vi "lantronix_discovery.vi"(8 "error in (no error)":errorcluster, 10 "timeout [ms] (1000)":dbl=1.0 caption="timeout [ms]", 11 "Local IP (optional)":string) -> (0 "error out":errorcluster, 3 "DEVICES":T1(array[cluster]))   [LabVIEW 2016]
doc: "This VI scans network and tries to find all connected Lantronix X-Port devices.\nThe result is array of clusters of 4 elements (IP, MAC, ID, version).\nUser can enter valid Local IP Address or this vi tries to get local IP from system.\n\nJakub Parez ATEsystem s.r.o. 2017"
uses:
  <vilib>/Utility/error.llb/Error Cluster From Error Code.vi
  <vilib>/regexp/Match Regular Expression.xnode
  <vilib>/ErrorRing/Error Ring.xnode
panel:
  # "IP"
  # "MAC"
  # "ID"
  # "version"
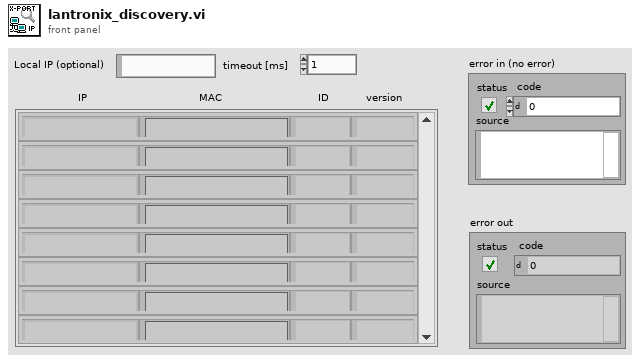
[diagram p1: front panel]
types:
  T1 = cluster{"IP":string, "MAC":string, "ID":string, "version":string}[]
  T2 = cluster{"IP":string, "MAC":string, "ID":string, "version":string}
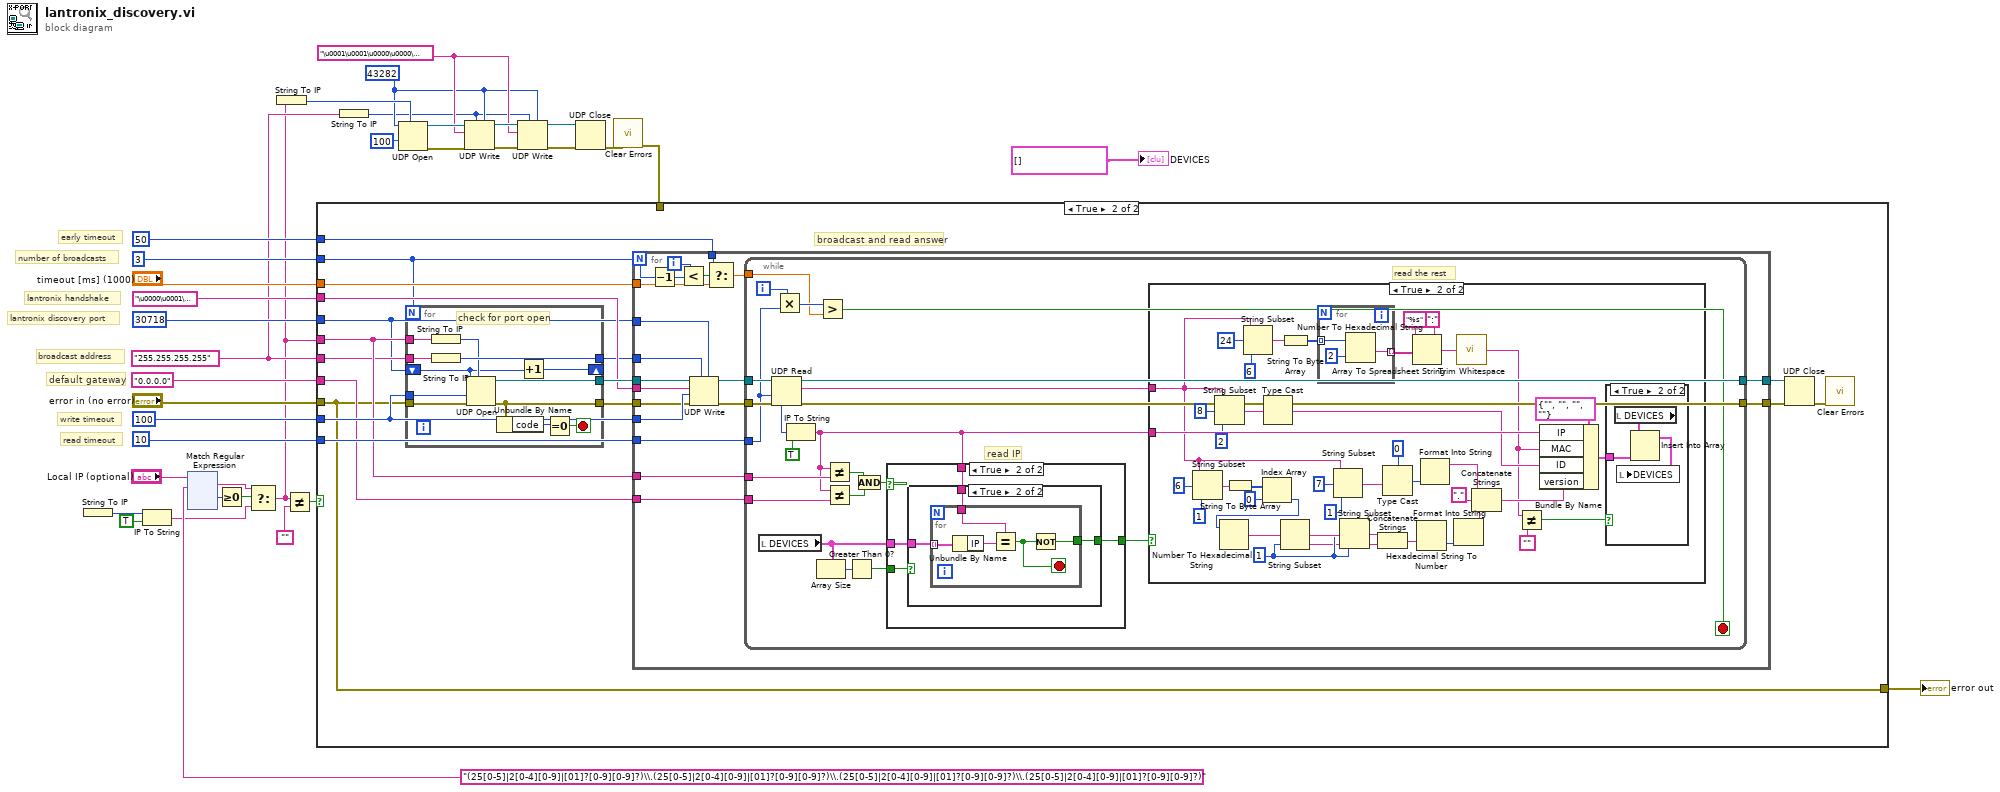
[diagram p0: block diagram]
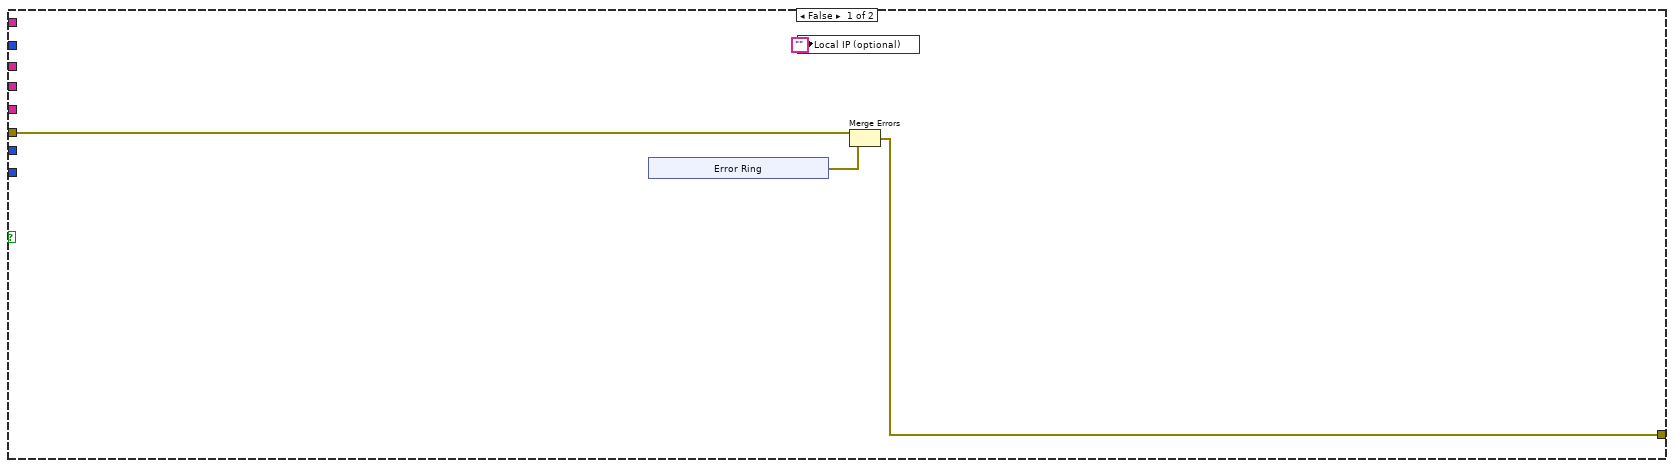
[diagram p2: hidden frame]
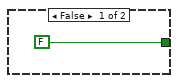
[diagram p3: hidden frame]
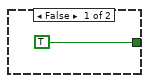
[diagram p4: hidden frame]
diagram:
  w14 = u16 43282 ("port")
  w15 = "\u0001\u0001\u0000\u0000\u0000ÿ\u0000\u0000" ("data in")
  w21 = "255.255.255.255"
  # "broadcast address"
  # "early timeout"
  # "default gateway"
  # "read timeout"
  # "write timeout"
  # "number of broadcasts"
  # "lantronix discovery port"
  # "lantronix handshake"
  n1 = String To IP() -> (0:w8:u32)  [unwired: 1 in]
  n2 = IP To String(1:TRUE ("dot notation? (F)"), 2:w8) -> (0:w4:string)
  n3 = xnode "Match Regular Expression"("input string"="Local IP (optional)", "regular expression"="(25[0-5]|2[0-4][0-9]|[01]?[0-9][0-9]?)\\.(25[0-5]|2[0-4][0-9]|[01]?[0-9][0-9]?)\\.(25[0-5]|2[0-4][0-9]|[01]?[0-9][0-9]?)\\.(25[0-5]|2[0-4][0-9]|[01]?[0-9][0-9]?)") -> ("whole match"=w5:string, "offset past match"=w27:i32)  [unwired: 4 in, 3 out]
  n4 = Greater Or Equal To 0?(x=w27) -> (x >= 0?=w6:bool)
  n5 = Select(t=w5, s=w6, f=w4) -> (s? t:f=w1:string)
  n6 = String To IP(1:w1) -> (0:w22:u32)
  n7 = Not Equal?(x=w1, y="") -> (x != y?=w2:bool)
  n8 = String To IP(1:w21) -> (0:w13:u32)
  n9 = UDP Open(7:w22, 9:100 ("timeout ms (25000)"), 11:w14) -> (port=w25:refnum<k16>, 0:w23:errorcluster)  [unwired: 2 in, 1 out]
  n10 = UDP Write(address=w13, port or service name=w14, connection ID=w25, data in=w15, 8:w23) -> (error out=w19:errorcluster, 3:w16:refnum<k16>)  [unwired: 1 in]
  n11 = UDP Write(address=w13, port or service name=w14, connection ID=w16, data in=w15, 8:w19) -> (error out=w18:errorcluster, 3:w17:refnum<k16>)  [unwired: 1 in]
  n12 = UDP Close(connection ID=w17, 8:w18) -> (error out=w24:errorcluster)  [unwired: 1 out]
  n13 = call <vilib>:"Clear Errors.vi"("error in (no error)"=w24) -> ("error out"=w20:errorcluster)  [unwired: 5 in, 1 out]
  n14 = case shown="True" w2 {
    tunnel: u16 10 ("port") -> [_ w60]
    tunnel: 100 ("timeout ms (25000)") -> [_ w59]
    tunnel: "\u0000\u0001\u0000ö" ("data in") -> [_ w56]
    tunnel: u16 30718 ("port") -> [_ w48]
    tunnel: "0.0.0.0" ("service name") -> [_ w55]
    tunnel: "timeout [ms] (1000)" -> [_ w54]
    tunnel: "error in (no error)" -> [w39 w46]
    tunnel: 3 ("timeout ms (25000)") -> [_ w47]
    tunnel: 50 ("timeout ms (25000)") -> [_ w52]
    tunnel: w1 -> [_ w50]
    tunnel: w21 -> [_ w49]
    tunnel: w20 -> [_ _]
    tunnel: [w37 w46] -> w9
    frame False {
      n15 = xnode "Error Ring"() -> ("error out"=w38:errorcluster)
      n16 = local write "Local IP (optional)"("") -> ()
      n17 = Merge Errors(w39, w38) -> (w37:errorcluster)
    }
    frame True {
      # "broadcast and read answer"
      n18 = for {
        N: w47 -> [_]
        tunnel: w59 -> [w74]
        tunnel: [w73] -> w58
        tunnel: [w71] -> w51
        tunnel: w50 -> [w70]
        tunnel: w49 -> [w69]
        tunnel: w46 -> [w72]
        tunnel: [w67] -> w57
        shift-right: [w63] -> _
        shift-left: w48 -> [w64]
        stop <- w65 stop-if-true
        # "check for port open"
        n19 = String To IP(1:w70) -> (0:w68:u32)
        n20 = String To IP(1:w69) -> (0:w71:u32)
        n21 = UDP Open(7:w68, 8:w72, 9:w74, 11:w64) -> (port=w73:refnum<k16>, 0:w67:errorcluster)  [unwired: 1 in, 1 out]
        n22 = Unbundle By Name(w67) -> ("code"=w66:i32)
        n23 = Increment(x=w64) -> (x+1=w63:u16)
        n24 = Equal To 0?(x=w66) -> (x = 0?=w65:bool)
      }
      n25 = for {
        N: w47 -> [w82]
        tunnel: w60 -> [w92]
        tunnel: w59 -> [w91]
        tunnel: w56 -> [w88]
        tunnel: w48 -> [w87]
        tunnel: w55 -> [w84]
        tunnel: w50 -> [w83]
        tunnel: w54 -> [w77]
        tunnel: w52 -> [w78]
        tunnel: w58 -> [w90]
        tunnel: [w94] -> w62
        tunnel: w57 -> [w89]
        tunnel: [w93] -> w61
        tunnel: w51 -> [w75]
        i -> [w81]
        n26 = Decrement(x=w82) -> (x-1=w80:i32)
        n27 = Less?(x=w81, y=w80) -> (x < y?=w79:bool)
        n28 = UDP Write(address=w75, port or service name=w87, connection ID=w90, data in=w88, 8:w89, 9:w91) -> (error out=w85:errorcluster, 3:w86:refnum<k16>)
        n29 = Select(t=w78, s=w79, f=w77) -> (s? t:f=w76:dbl)
        n30 = while {
          tunnel: w92 -> [w109]
          tunnel: w86 -> [w116]
          tunnel: [w115] -> w94
          tunnel: w85 -> [w114]
          tunnel: [w113] -> w93
          tunnel: w83 -> [w111]
          tunnel: w84 -> [w110]
          tunnel: w76 -> [w105]
          i -> [w108]
          stop <- w106 stop-if-true
          # "read the rest"
          # "read IP"
          n31 = local read "DEVICES"() -> (w101:T1)
          n32 = UDP Read(connection ID=w116, timeout ms (25000)=w109, 8:w114) -> (data out=w95:string, error out=w113:errorcluster, 3:w115:refnum<k16>, 6:w97:u32)  [unwired: 1 in, 1 out]
          n33 = Multiply(x=w108, y=w109) -> (x*y=w107:i32)
          n34 = IP To String(1:TRUE ("dot notation? (F)"), 2:w97) -> (0:w96:string)
          n35 = Array Size(array=w101) -> (size(s)=w100:i32)
          n36 = Greater?(x=w107, y=w105) -> (0:w106:bool)
          n37 = Not Equal?(x=w96, y=w111) -> (x != y?=w104:bool)
          n38 = Not Equal?(x=w96, y=w110) -> (x != y?=w103:bool)
          n39 = Greater Than 0?(x=w100) -> (x > 0?=w99:bool)
          n40 = And(x=w104, y=w103) -> (x .and. y?=w102:bool)
          n41 = case shown="True" w102 {
            tunnel: w96 -> [_ w121]
            tunnel: [FALSE w118] -> w98
            tunnel: w101 -> [_ w120]
            tunnel: w99 -> [_ w119]
            frame False {
            }
            frame True {
              n42 = case shown="True" w119 {
                tunnel: w121 -> [_ w125]
                tunnel: w120 -> [_ w124]
                tunnel: [TRUE w123] -> w118
                frame False {
                }
                frame True {
                  n43 = for {
                    tunnel: w124 -> [w130] mode=indexing
                    tunnel: w125 -> [w128]
                    tunnel: [w126] -> w123
                    stop <- w127 stop-if-true
                    n44 = Unbundle By Name(w130) -> ("IP"=w129:string)
                    n45 = Equal?(x=w128, y=w129) -> (x = y?=w127:bool)
                    n46 = Not(x=w127) -> (.not. x?=w126:bool)
                  }
                }
              }
            }
          }
          n47 = case shown="True" w98 {
            tunnel: w96 -> [_ w168]
            tunnel: w95 -> [_ w153]
            frame False {
            }
            frame True {
              w140 = 1 ("offset (0)")
              n48 = String Subset(string=w153, offset (0)=6 ("length (rest)"), length (rest)=1 ("length (rest)")) -> (substring=w145:string)
              n49 = String Subset(string=w153, offset (0)=8 ("length (rest)"), length (rest)=2 ("length (rest)")) -> (substring=w158:string)
              n50 = String To Byte Array(string=w145) -> (unsigned byte array=w144:u8[])
              n51 = String Subset(string=w153, offset (0)=24 ("length (rest)"), length (rest)=6 ("length (rest)")) -> (substring=w166:string)
              n52 = Index Array(array=w144, index=0) -> (element=w142:u8)
              n53 = Number To Hexadecimal String(2:w142) -> (0:w141:string)  [unwired: 1 in]
              n54 = Type Cast(x=w158) -> (*(type *) &x=w157:string)  [unwired: 1 in]
              n55 = String Subset(string=w141, length (rest)=w140) -> (substring=w137:string)  [unwired: 1 in]
              n56 = String To Byte Array(string=w166) -> (unsigned byte array=w165:u8[])
              n57 = for {
                tunnel: w165 -> [w176] mode=indexing
                tunnel: [w174] -> w164 mode=indexing
                n58 = Number To Hexadecimal String(1:i16 2 ("width (-)"), 2:w176) -> (0:w174:string)
              }
              n59 = String Subset(string=w153, offset (0)=7 ("length (rest)"), length (rest)=1 ("length (rest)")) -> (substring=w151:string)
              n60 = String Subset(string=w141, offset (0)=w140, length (rest)=w140) -> (substring=w138:string)
              n61 = Concatenate Strings(w138, w137) -> (w136:string)
              n62 = Type Cast(type=u8 0 ("y"), x=w151) -> (*(type *) &x=w149:u8)
              n63 = Array To Spreadsheet String(delimiter (Tab)=":", array=w164, 3:"%s" ("format string")) -> (spreadsheet string=w134:string)
              n64 = Hexadecimal String To Number(string=w136) -> (number=w135:u32)  [unwired: 2 in, 1 out]
              n65 = Format Into String(w149) -> (resulting string=w148:string)  [unwired: 3 in, 1 out]
              n66 = Format Into String(w135) -> (resulting string=w147:string)  [unwired: 3 in, 1 out]
              n67 = call <vilib>:"Trim Whitespace.vi"("string"=w134) -> ("trimmed string"=w133:string)  [unwired: 1 in]
              n68 = Concatenate Strings(w148, "." ("f"), w147) -> (w146:string)
              n69 = Not Equal?(x=w133, y="") -> (x != y?=w131:bool)
              n70 = Bundle By Name(cluster=T2 {"IP"="", "MAC"="", "ID"="", "version"=""}, "IP"=w168, "MAC"=w133, "ID"=w157, "version"=w146) -> (w170:T2)
              n71 = case shown="True" w131 {
                tunnel: w170 -> [_ w172]
                frame False {
                }
                frame True {
                  n72 = local read "DEVICES"() -> (w171:T1)
                  n73 = Insert Into Array(array=w171, new element=w172) -> (w173:T1)  [unwired: 1 in]
                  n74 = local write "DEVICES"(w173) -> ()
                }
              }
            }
          }
        }
      }
      n75 = UDP Close(connection ID=w62, 8:w61) -> (error out=w53:errorcluster)  [unwired: 1 out]
      n76 = call <vilib>:"Clear Errors.vi"("error in (no error)"=w53) -> ()  [unwired: 5 in, 2 out]
    }
  }
  "error out" <- w9
  "DEVICES" <- T1 []
